vi "requeteBDD.vi"(1 "Requête Sql":string) -> (0 "Table Control":string[][](table))   [LabVIEW 2024]
uses:
  <vilib>/drjdpowell/SQLite Library/SQL Connection/Open (string).vi
  <vilib>/drjdpowell/SQLite Library/SQL Connection/Execute SQL.vi
  <vilib>/drjdpowell/SQLite Library/SQL Connection/Connection.lvclass
  <vilib>/drjdpowell/SQLite Library/SQLite.lvlib
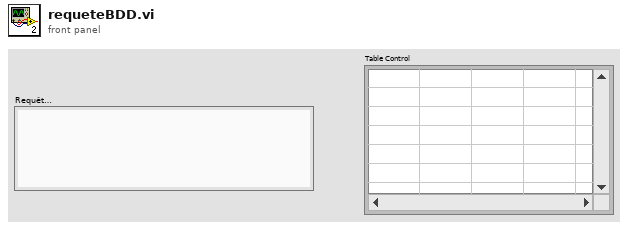
[diagram p1: front panel]
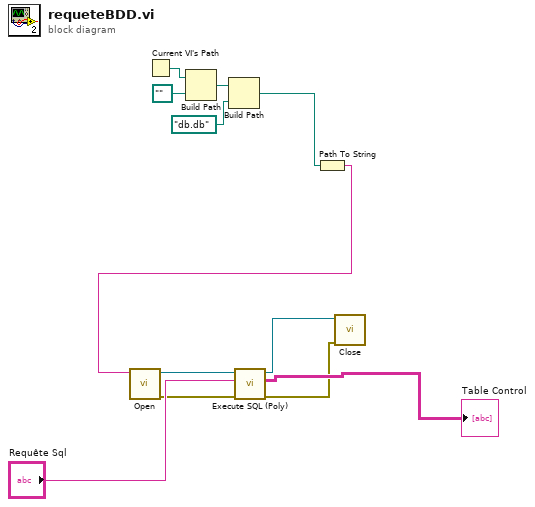
[diagram p0: block diagram]
diagram:
  n1 = Current VI's Path() -> (path=w6:path)
  n2 = Build Path(base path=w6, name or relative path=path "..") -> (appended path=w3:path)
  n3 = Build Path(base path=w3, name or relative path=path "db.db" ("Filename")) -> (appended path=w2:path)
  n4 = Path To String(path=w2) -> (string=w1:string)
  n5 = call-poly <vilib>:"Open.vi"("db file"=w1) -> ("error out"=w9:errorcluster, "SQLite Connection"=w12:refnum<class "Connection.lvclass">)  [unwired: 9 in]
  n6 = call-poly <vilib>:"Execute SQL (Poly).vi"("error in (no error)"=w9, "SQL"="Requête Sql", "SQLite Connection in"=w12) -> ("error out"=w8:errorcluster, "Result Set"=→"Table Control":string[][], "SQLite Connection"=w7:refnum<class "Connection.lvclass">)  [unwired: 5 in, 1 out]
  n7 = call-dynamic "Close.vi"("error in (no error)"=w8, "SQLite Connection in"=w7) -> ()  [unwired: 9 in, 1 out]
